vi "TCP_check.vi"() -> ()   [LabVIEW 2015]
panel:
  out "data out":string
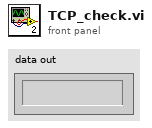
[diagram p1: front panel]
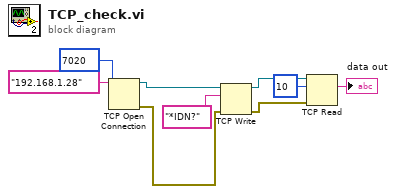
[diagram p0: block diagram]
diagram:
  n1 = TCP Open Connection(address="192.168.1.28", remote port or service name=u16 7020) -> (connection ID=w7:refnum<k5>, error out=w5:errorcluster)  [unwired: 3 in]
  n2 = TCP Write(connection ID=w7, data in="*IDN?", error in (no error)=w5) -> (connection ID out=w3:refnum<k5>, error out=w4:errorcluster)  [unwired: 1 in, 1 out]
  n3 = TCP Read(connection ID=w3, bytes to read=10, error in (no error)=w4) -> (data out=→"data out":string)  [unwired: 2 in, 2 out]
